vi "Choose Shot Type.vi"(11 "Manipulator D-Pad":T2) -> (3 "Shot Type":T1)   [LabVIEW 2015]
uses:
  Common Code/Gamepads/D-Pad.ctl
  Common Code/Shot Type.ctl
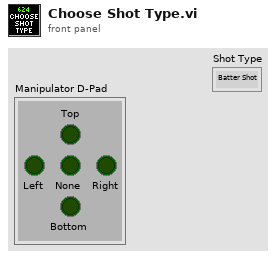
[diagram p1: front panel]
types:
  T1 = typedef "Shot Type.ctl" = enum16{"Batter Shot", "Corner Shot", "Cleat Shot", "Vision Shot", "Deep Middle Shot"}
  T2 = typedef "D-Pad.ctl" = cluster{"Top":bool, "Bottom":bool, "None":bool, "Right":bool, "Left":bool}
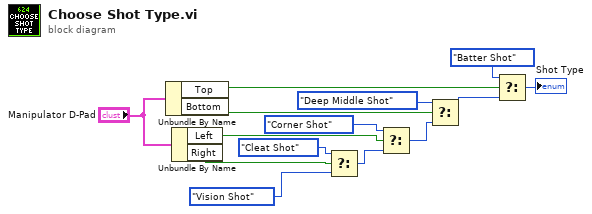
[diagram p0: block diagram]
diagram:
  n1 = Unbundle By Name("Manipulator D-Pad") -> ("Top"=w2:bool, "Bottom"=w4:bool)
  n2 = Unbundle By Name("Manipulator D-Pad") -> ("Left"=w8:bool, "Right"=w11:bool)
  n3 = Select(t=Shot_Type."Cleat Shot" ("Shot Type"), s=w11, f=Shot_Type."Vision Shot" ("Shot Type")) -> (s? t:f=w13:T1)
  n4 = Select(t=Shot_Type."Corner Shot" ("Shot Type"), s=w8, f=w13) -> (s? t:f=w10:T1)
  n5 = Select(t=Shot_Type."Deep Middle Shot" ("Shot Type"), s=w4, f=w10) -> (s? t:f=w6:T1)
  n6 = Select(t=Shot_Type."Batter Shot" ("Shot Type"), s=w2, f=w6) -> (s? t:f=→"Shot Type":T1)
